vi "niWLAN - 80211abgnIQMeasurementsSettings.vi"(0 "niwlan analysis session":T6, 1 "WLAN Measurement Settings":T1={"OFDM Advanced Controls(11ag)"={"OFDM Auto Compute Acquisition Length Enabled"=0, "OFDM Maximum Symbols Used"=0, "OFDM Time Tracking Enabled"=0, "OFDM Channel Tracking Enabled"=0, "OFDM Amplitude Tracking Enabled"=1, "OFDM CFO Estimation Method"=0, "OFDM Phase Tracking Method"=0, "OFDM Header Detection Enabled"=0, "OFDM MAC FCS Check Enabled"=0, "#Avg"=10, "#Iterations"=10}, "DSSS Demod Parameters"={"DSSS Auto Compute Acquisition Length Enabled"=0, "DSSS Equalization Enabled"=0, "DSSS Header Detection Enabled"=0, "DSSS MAC FCS Check Enabled"=0, "DSSS Measurement Start Location"=0, "DSSS Phase Tracking Method"=0, "DSSS Maximum Chips Used"=0, "DSSS Reference Pulse Shaping Filter"=0, "DSSS Reference Pulse Shaping Filter Coefficient"=0.0, "# Avg"=1024, "# Iterations"=1024, "DSSS Power Ramp Enabled"=0}, "OFDM Advanced Controls (11n)"={"OFDM Auto Compute Acquisition Length Enabled"=0, "OFDM Maximum Symbols Used"=0, "OFDM Time Tracking Enabled"=0, "OFDM Channel Tracking Enabled"=0, "OFDM Amplitude Tracking Enabled"=1, "OFDM CFO Estimation Method"=0, "OFDM Phase Tracking Method"=0, "OFDM Header Detection Enabled"=0, "OFDM MAC FCS Check Enabled"=0, "#Avg"=10, "#Iterations"=10}, "OFDM Advanced Controls(11ac)"={"OFDM Auto Compute Acquisition Length Enabled"=0, "OFDM Maximum Symbols Used"=0, "OFDM Time Tracking Enabled"=1, "OFDM Channel Tracking Enabled"=0, "OFDM Amplitude Tracking Enabled"=0, "OFDM CFO Estimation Method"=0, "OFDM Phase Tracking Method"=0, "OFDM Header Detection Enabled"=0, "OFDM MAC FCS Check Enabled"=0, "#Avg"=10, "#Iterations"=10}} {"OFDM Advanced Controls(11ac)"."OFDM Phase Tracking Method" items=["Standard", "Instantaneous", "None", "Standard with Cubic Spline Fit"]; "OFDM Advanced Controls(11ac)"."OFDM CFO Estimation Method" items=["Preamble Only", "Preamble and Data"]; "OFDM Advanced Controls(11ac)"."OFDM Channel Tracking Enabled" items=["False", "True"]; "OFDM Advanced Controls(11ac)"."OFDM Amplitude Tracking Enabled" items=["False", "True"]; "OFDM Advanced Controls(11ac)"."OFDM Time Tracking Enabled" items=["True"=1, "False"=0]; "OFDM Advanced Controls(11ac)"."OFDM Auto Compute Acquisition Length Enabled" items=["False", "True"]; "OFDM Advanced Controls(11ac)"."OFDM MAC FCS Check Enabled" items=["False", "True"]; "OFDM Advanced Controls(11ac)"."OFDM Header Detection Enabled" items=["False", "True"]; "OFDM Advanced Controls (11n)"."OFDM Phase Tracking Method" items=["Standard", "Instantaneous", "None", "Standard with Cubic Spline Fit"]; "OFDM Advanced Controls (11n)"."OFDM CFO Estimation Method" items=["Preamble Only", "Preamble and Data"]; "OFDM Advanced Controls (11n)"."OFDM Channel Tracking Enabled" items=["False", "True"]; "OFDM Advanced Controls (11n)"."OFDM Amplitude Tracking Enabled" items=["False", "True"]; "OFDM Advanced Controls (11n)"."OFDM Time Tracking Enabled" items=["True"=1, "False"=0]; "OFDM Advanced Controls (11n)"."OFDM Auto Compute Acquisition Length Enabled" items=["False", "True"]; "OFDM Advanced Controls (11n)"."OFDM MAC FCS Check Enabled" items=["False", "True"]; "OFDM Advanced Controls (11n)"."OFDM Header Detection Enabled" items=["False", "True"]; "DSSS Demod Parameters"."DSSS Power Ramp Enabled" items=["False", "True"]; "DSSS Demod Parameters"."DSSS Auto Compute Acquisition Length Enabled" items=["False", "True"]; "DSSS Demod Parameters"."DSSS Phase Tracking Method" items=["Standard", "Instantaneous"]; "DSSS Demod Parameters"."DSSS Equalization Enabled" items=["False", "True"]; "DSSS Demod Parameters"."DSSS Reference Pulse Shaping Filter" items=["Rectangular", "Raised Cosine", "Root Raised Cosine", "Gaussian"]; "DSSS Demod Parameters"."DSSS MAC FCS Check Enabled" items=["False", "True"]; "DSSS Demod Parameters"."DSSS Header Detection Enabled" items=["False", "True"]; "OFDM Advanced Controls(11ag)"."OFDM Phase Tracking Method" items=["Standard", "Instantaneous", "None", "Standard with Cubic Spline Fit"]; "OFDM Advanced Controls(11ag)"."OFDM CFO Estimation Method" items=["Preamble Only", "Preamble and Data"]; "OFDM Advanced Controls(11ag)"."OFDM Channel Tracking Enabled" items=["False", "True"]; "OFDM Advanced Controls(11ag)"."OFDM Amplitude Tracking Enabled" items=["False", "True"]; "OFDM Advanced Controls(11ag)"."OFDM Time Tracking Enabled" items=["True"=1, "False"=0]; "OFDM Advanced Controls(11ag)"."OFDM Auto Compute Acquisition Length Enabled" items=["False", "True"]; "OFDM Advanced Controls(11ag)"."OFDM MAC FCS Check Enabled" items=["False", "True"]; "OFDM Advanced Controls(11ag)"."OFDM Header Detection Enabled" items=["False", "True"]}, 2 "Measurement Type":T4(ring), 5 "TV Parameters(DataType)":T5 {"Standard" items=["80211A/G/J/P OFDM", "80211B/G DSSS", "80211G DSSSOFDM", "80211N MIMOOFDM", "80211AC MIMOOFDM"]; "OFDM Data Rate (Mbps)" items=["6", "9", "12", "18", "24", "36", "48", "54"]; "80211n PLCP Frame Format" items=["Mixed Format", "Greenfield Format"]; "FEC Coding Type" items=["BCC", "LDPC"]; "DSSS Data Rate (Mbps)" items=["1", "2", "5.5 CCK", "5.5 PBCC", "11 CCK", "11 PBCC", "22", "33"]}, 7 "Set TV ?":bool, 11 "error in":errorcluster, 13 "Cal Routine ?":bool) -> (4 "niWLAN session":T6, 15 "error out":errorcluster)   [LabVIEW 2012]
uses:
  <vilib>/RF Toolkits/WLAN/analysis/controls/wlanv1 Analysis Refnum.ctl
  TV/RW/Includes/WLAN - TV - RW - INC - TV_DataType_Cluster.ctl
  TV/RW/Includes/WLAN - TV - RW - INC - Tx_Measurement_Cluster.ctl
  TV/RW/Includes/WLAN - TV - RW - INC - TV_OFDM Demod.ctl
  TV/RW/Includes/WLAN - TV - RW - INC - TV_DSSS Demod.ctl
  <resource>/objmgr/niWLANAnalysis.rc
panel:
  out "Standard":i32(ring) items=["80211A/G/J/P OFDM", "80211B/G DSSS", "80211G DSSSOFDM", "80211N MIMOOFDM", "80211AC MIMOOFDM"]
  # "Hardware Configuration"
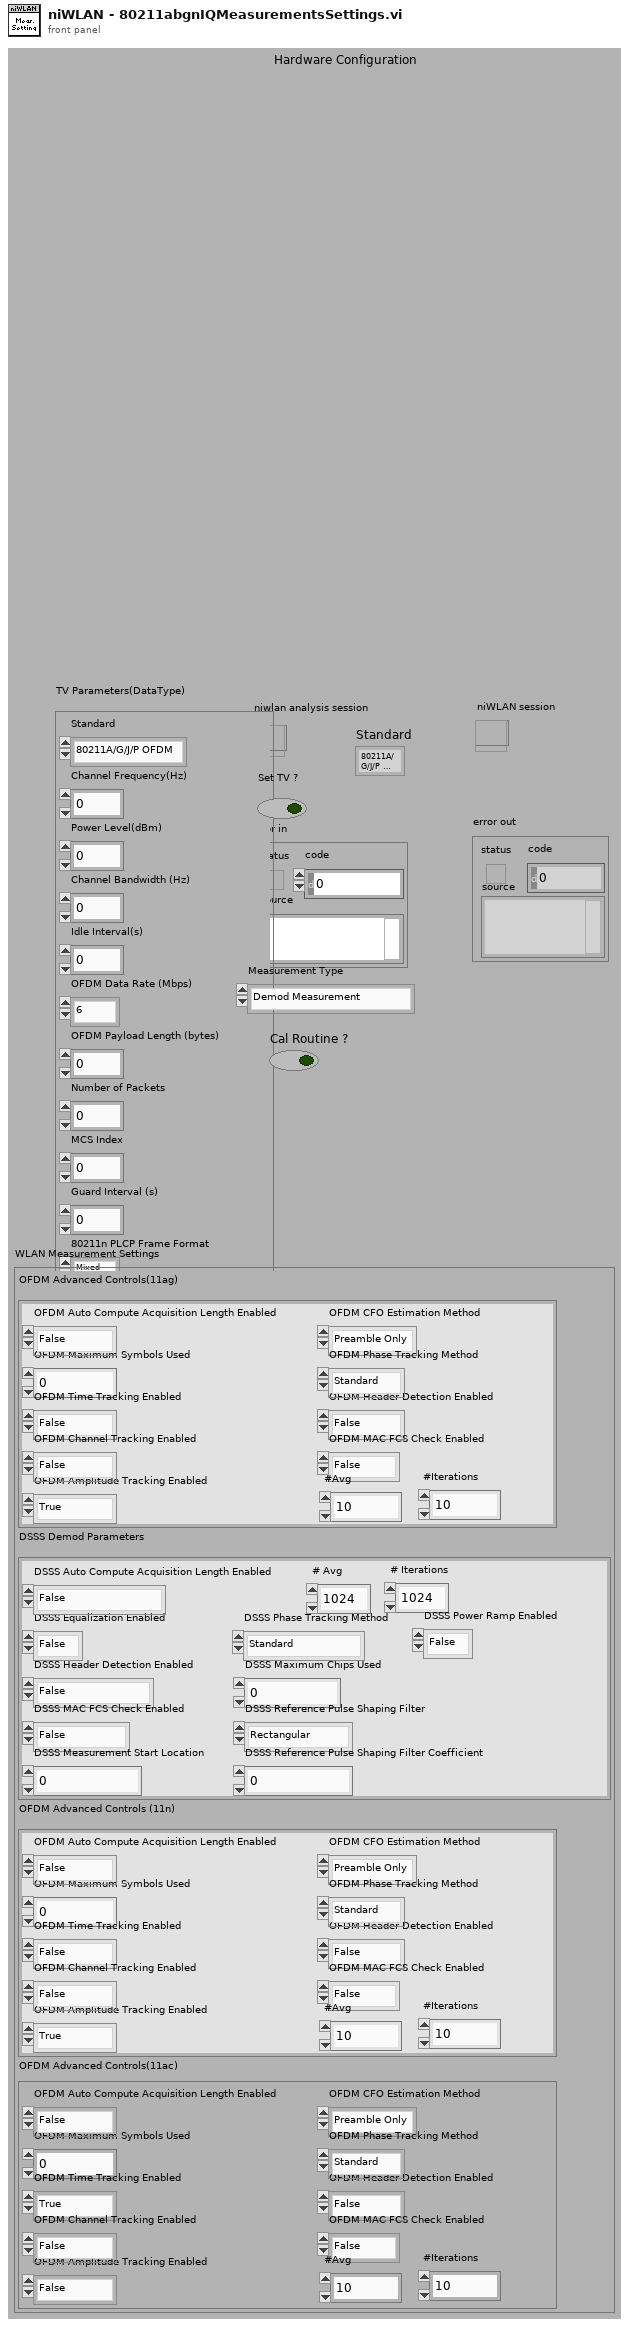
[diagram p1: front panel]
types:
  T1 = typedef "WLAN - TV - RW - INC - Tx_Measurement_Cluster.ctl" = cluster{"OFDM Advanced Controls(11ag)":T2, "DSSS Demod Parameters":T3, "OFDM Advanced Controls (11n)":T2, "OFDM Advanced Controls(11ac)":cluster{"OFDM Auto Compute Acquisition Length Enabled":i32, "OFDM Maximum Symbols Used":i32, "OFDM Time Tracking Enabled":i32, "OFDM Channel Tracking Enabled":i32, "OFDM Amplitude Tracking Enabled":i32, "OFDM CFO Estimation Method":i32, "OFDM Phase Tracking Method":i32, "OFDM Header Detection Enabled":i32, "OFDM MAC FCS Check Enabled":i32, "#Avg":i32, "#Iterations":i32}}
  T2 = typedef "WLAN - TV - RW - INC - TV_OFDM Demod.ctl" = cluster{"OFDM Auto Compute Acquisition Length Enabled":i32, "OFDM Maximum Symbols Used":i32, "OFDM Time Tracking Enabled":i32, "OFDM Channel Tracking Enabled":i32, "OFDM Amplitude Tracking Enabled":i32, "OFDM CFO Estimation Method":i32, "OFDM Phase Tracking Method":i32, "OFDM Header Detection Enabled":i32, "OFDM MAC FCS Check Enabled":i32, "#Avg":i32, "#Iterations":i32}
  T3 = typedef "WLAN - TV - RW - INC - TV_DSSS Demod.ctl" = cluster{"DSSS Auto Compute Acquisition Length Enabled":i32, "DSSS Equalization Enabled":i32, "DSSS Header Detection Enabled":i32, "DSSS MAC FCS Check Enabled":i32, "DSSS Measurement Start Location":i32, "DSSS Phase Tracking Method":i32, "DSSS Maximum Chips Used":i32, "DSSS Reference Pulse Shaping Filter":i32, "DSSS Reference Pulse Shaping Filter Coefficient":dbl, "# Avg":i32, "# Iterations":i32, "DSSS Power Ramp Enabled":i32}
  T4 = enum16{"Demod Measurement", "Spectrum Measurement"}
  T5 = typedef "WLAN - TV - RW - INC - TV_DataType_Cluster.ctl" = cluster{"Standard":i32, "Channel Frequency(Hz)":dbl, "Power Level(dBm)":dbl, "Channel Bandwidth (Hz)":dbl, "Idle Interval(s)":dbl, "OFDM Data Rate (Mbps)":i32, "OFDM Payload Length (bytes)":i32, "Number of Packets":i32, "MCS Index":i32, "Guard Interval (s)":dbl, "80211n PLCP Frame Format":i32, "FEC Coding Type":i32, "DSSS Data Rate (Mbps)":i32, "DSSS Payload Length (bytes)":i32, "N_SS":i32}
  T6 = typedef "wlanv1 Analysis Refnum.ctl" = refnum<k20>
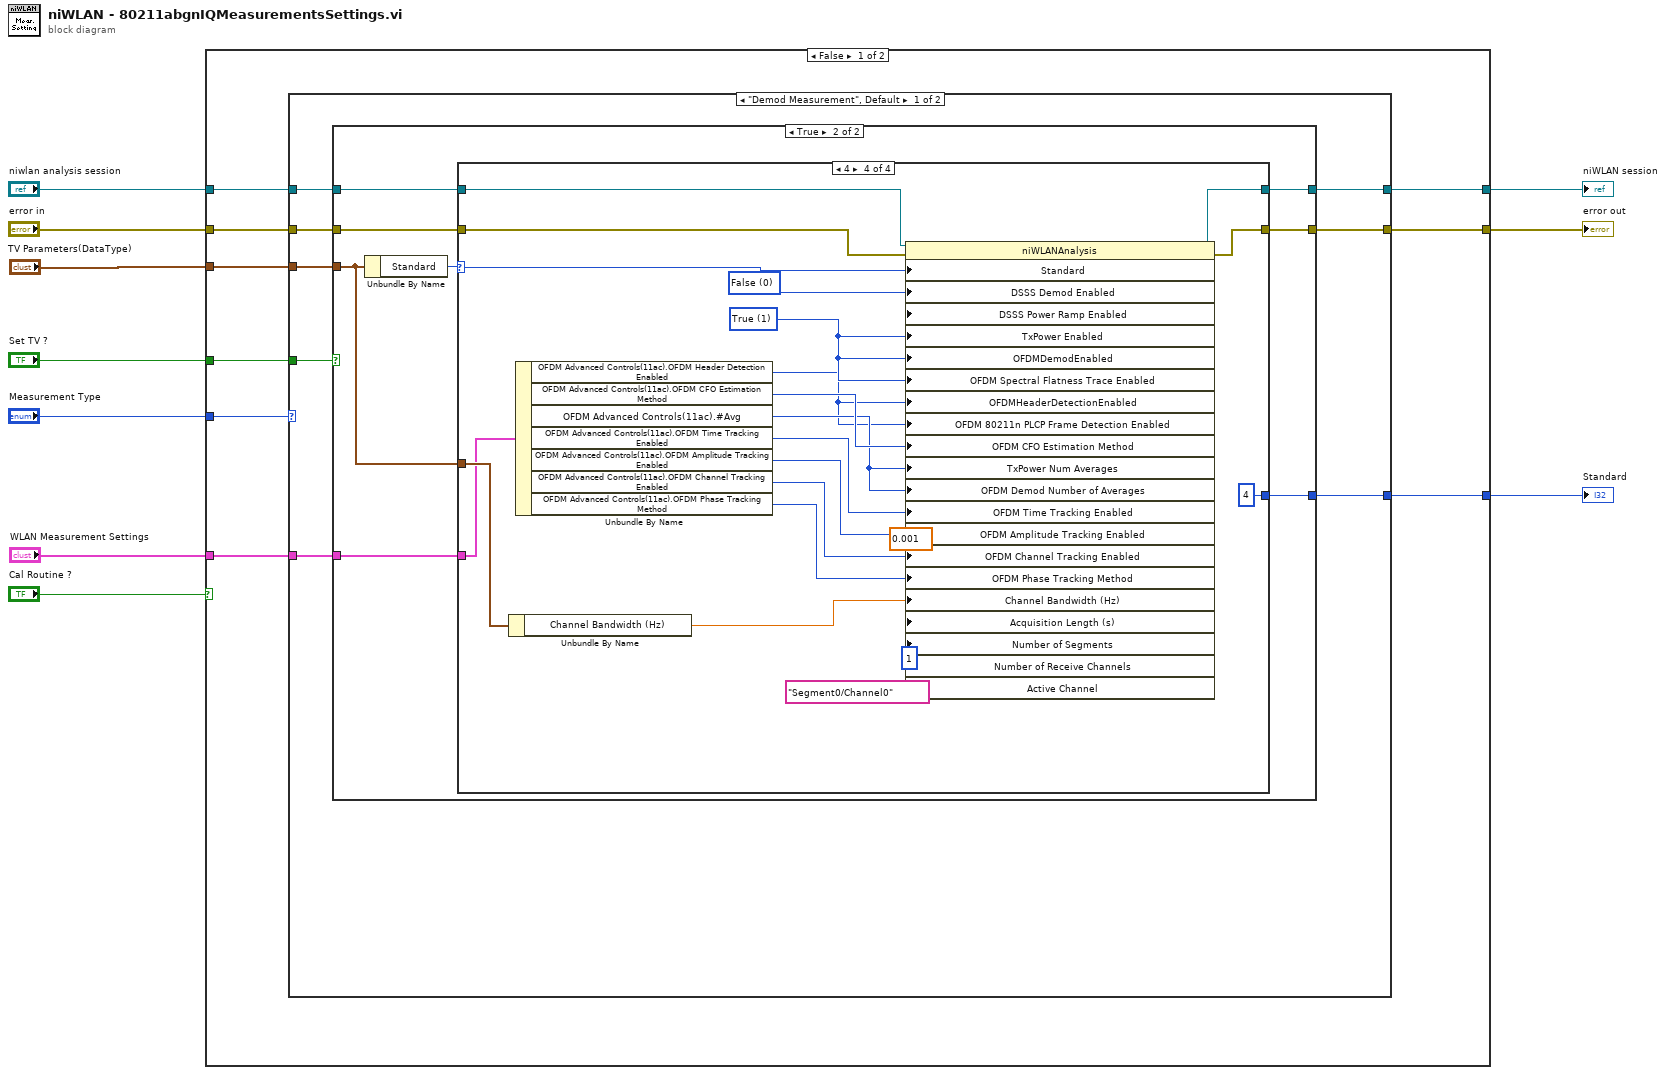
[diagram p0: block diagram]
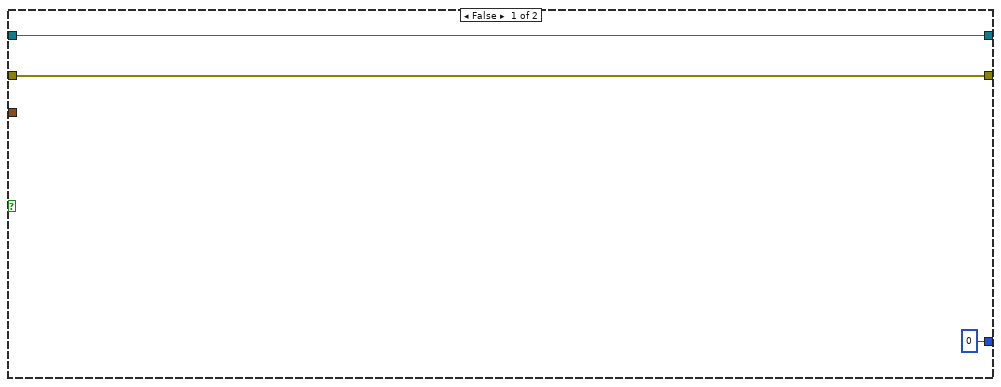
[diagram p2: hidden frame]
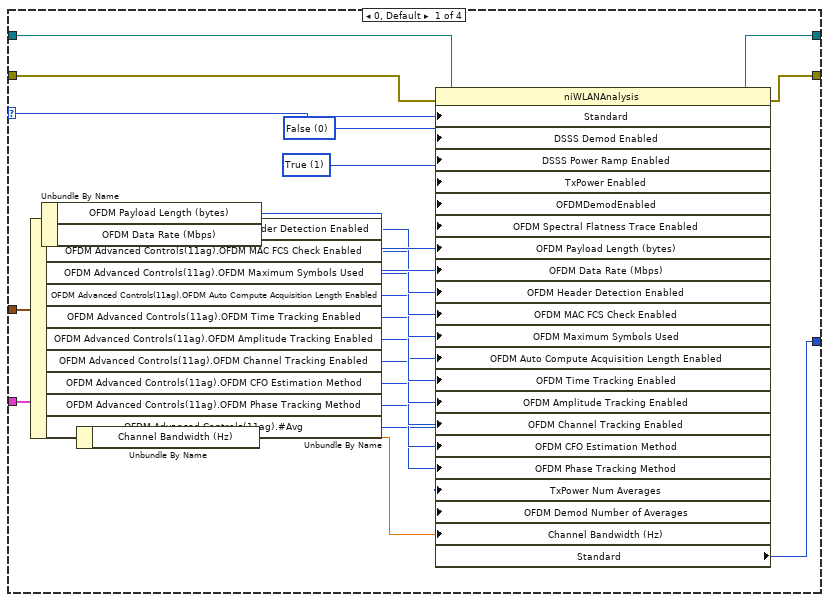
[diagram p3: hidden frame]
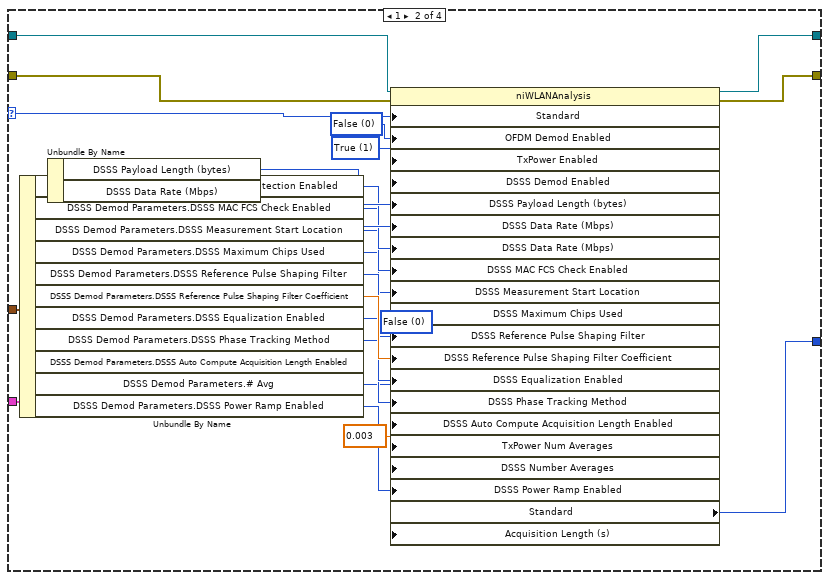
[diagram p4: hidden frame]
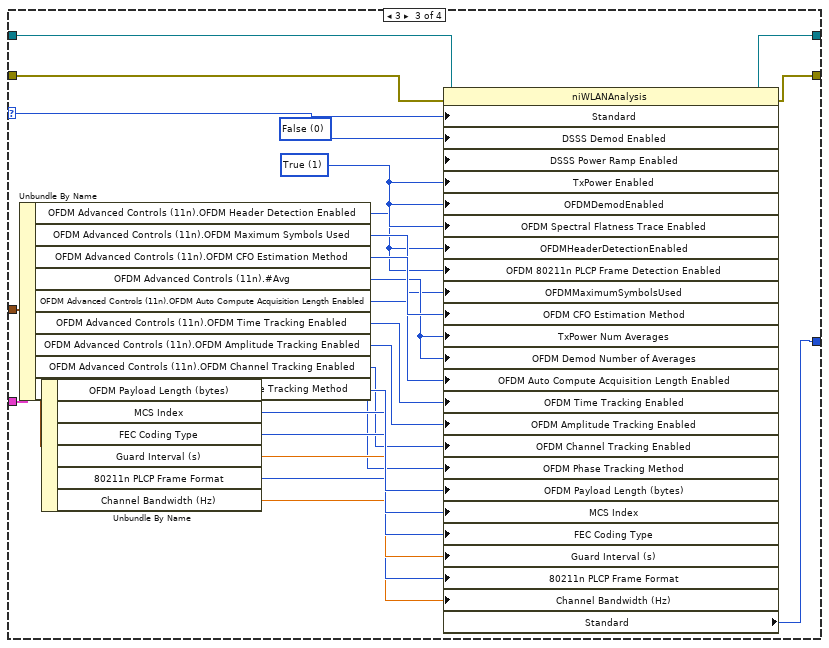
[diagram p5: hidden frame]
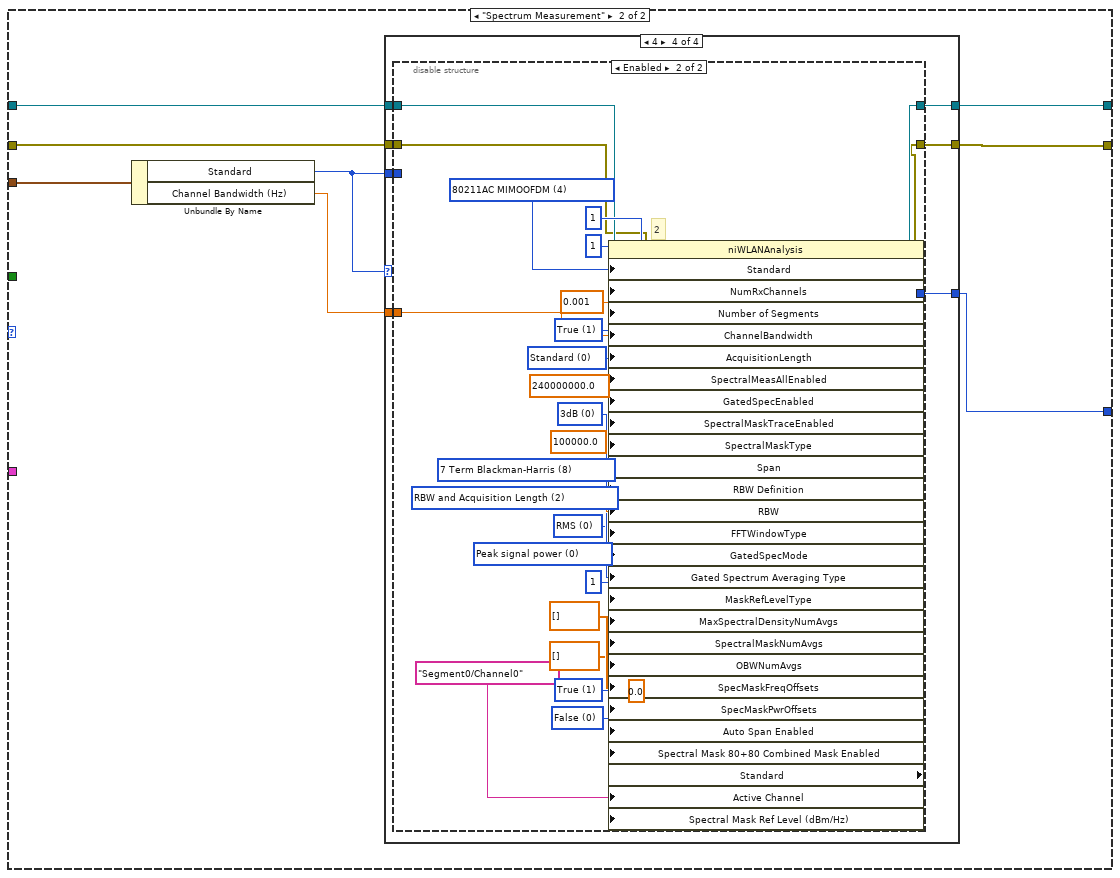
[diagram p6: hidden frame]
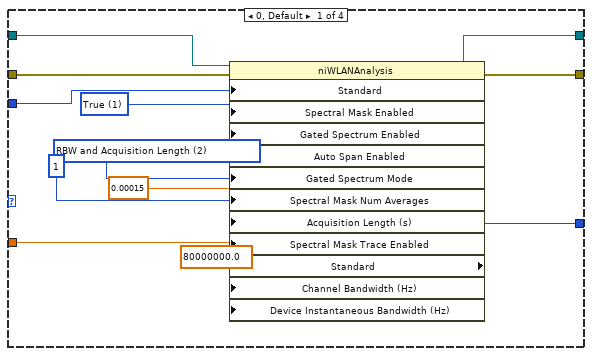
[diagram p7: hidden frame]
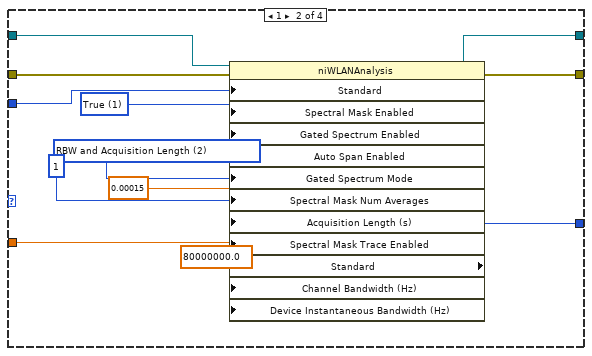
[diagram p8: hidden frame]
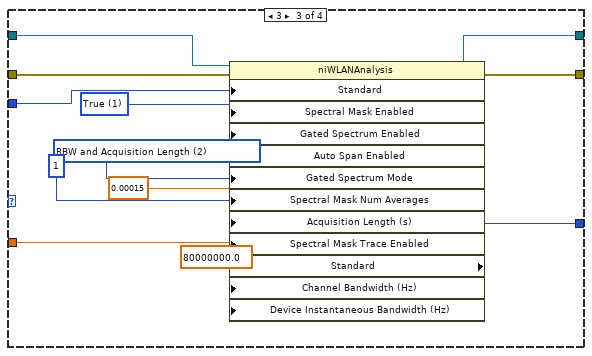
[diagram p9: hidden frame]
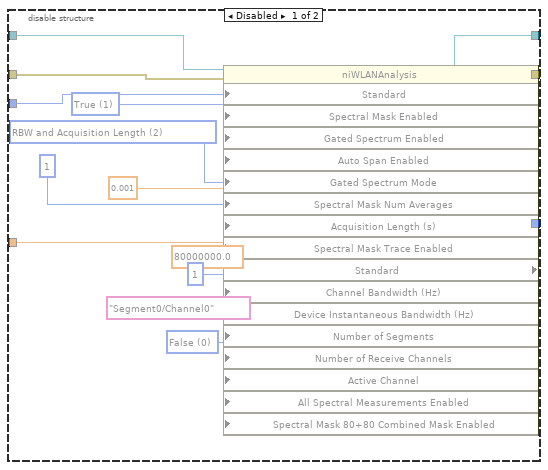
[diagram p10: hidden frame]
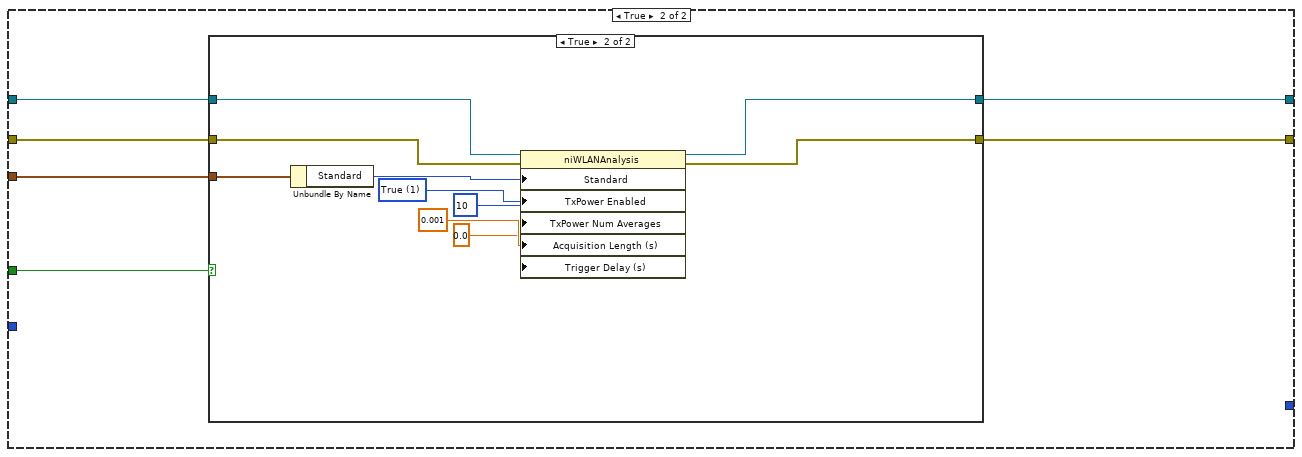
[diagram p11: hidden frame]
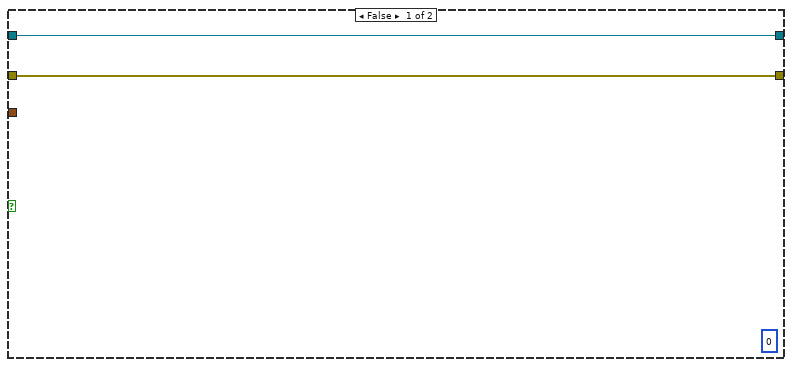
[diagram p12: hidden frame]
diagram:
  n1 = case shown="False" "Cal Routine ?" {
    tunnel: "niwlan analysis session" -> [w19 w229]
    tunnel: "error in" -> [w18 w228]
    tunnel: [w17 w227] -> w8
    tunnel: [w16 w226] -> w7
    tunnel: "TV Parameters(DataType)" -> [w15 w225]
    tunnel: "Set TV ?" -> [w14 w224]
    tunnel: "Measurement Type" -> [w13 _]
    tunnel: [w12 _] -> w3
    tunnel: "WLAN Measurement Settings" -> [w11 _]
    frame False {
      n2 = case shown="\"Demod Measurement\", Default" w13 {
        tunnel: w19 -> [w27 w139]
        tunnel: w18 -> [w26 w138]
        tunnel: [w25 w136] -> w17
        tunnel: [w24 w135] -> w16
        tunnel: w15 -> [w23 w137]
        tunnel: w14 -> [w22 _]
        tunnel: [w21 w134] -> w12
        tunnel: w11 -> [w20 _]
        frame "Demod Measurement", Default {
          n3 = case shown="True" w22 {
            tunnel: w27 -> [w30 w38]
            tunnel: w26 -> [w29 w37]
            tunnel: [w30 w36] -> w25
            tunnel: [w29 w35] -> w24
            tunnel: w23 -> [_ w33]
            tunnel: [0 ("Standard") w32] -> w21
            tunnel: w20 -> [_ w31]
            frame False {
            }
            frame True {
              n4 = Unbundle By Name(w33) -> ("Standard"=w34:i32)
              n5 = case shown="4" w34 {
                selector: w34 -> [w57 w81 w106 w127]
                tunnel: w38 -> [w61 w85 w110 w131]
                tunnel: w37 -> [w60 w84 w109 w130]
                tunnel: [w59 w83 w108 w129] -> w36
                tunnel: [w58 w82 w107 w128] -> w35
                tunnel: w33 -> [w43 w80 w105 w126]
                tunnel: [w41 w65 w98 4 ("Standard")] -> w32
                tunnel: w31 -> [w54 w75 w97 w124]
                frame 0, Default {
                  w39 = 0 items=["False", "True"] ("DSSS Demod Enabled")
                  w53 = 1 items=["False", "True"] ("OFDMDemodEnabled")
                  n6 = Unbundle By Name(w54) -> ("OFDM Advanced Controls(11ag).OFDM Header Detection Enabled"=w52:i32, "OFDM Advanced Controls(11ag).OFDM MAC FCS Check Enabled"=w51:i32, "OFDM Advanced Controls(11ag).OFDM Maximum Symbols Used"=w50:i32, "OFDM Advanced Controls(11ag).OFDM Auto Compute Acquisition Length Enabled"=w40:i32, "OFDM Advanced Controls(11ag).OFDM Time Tracking Enabled"=w49:i32, "OFDM Advanced Controls(11ag).OFDM Amplitude Tracking Enabled"=w48:i32, "OFDM Advanced Controls(11ag).OFDM Channel Tracking Enabled"=w47:i32, "OFDM Advanced Controls(11ag).OFDM CFO Estimation Method"=w46:i32, "OFDM Advanced Controls(11ag).OFDM Phase Tracking Method"=w45:i32, "OFDM Advanced Controls(11ag).#Avg"=w44:i32)
                  n7 = Unbundle By Name(w43) -> ("OFDM Payload Length (bytes)"=w56:i32, "OFDM Data Rate (Mbps)"=w55:i32)
                  n8 = Unbundle By Name(w43) -> ("Channel Bandwidth (Hz)"=w42:dbl)
                  n9 = property class="niWLANAnalysis"(reference=w61, error in=w60, "Standard"=w57, "DSSS Demod Enabled"=w39, "DSSS Power Ramp Enabled"=w39, "TxPower Enabled"=w53, "OFDMDemodEnabled"=w53, "OFDM Spectral Flatness Trace Enabled"=w53, "OFDM Payload Length (bytes)"=w56, "OFDM Data Rate (Mbps)"=w55, "OFDM Header Detection Enabled"=w52, "OFDM MAC FCS Check Enabled"=w51, "OFDM Maximum Symbols Used"=w50, "OFDM Auto Compute Acquisition Length Enabled"=w40, "OFDM Time Tracking Enabled"=w49, "OFDM Amplitude Tracking Enabled"=w48, "OFDM Channel Tracking Enabled"=w47, "OFDM CFO Estimation Method"=w46, "OFDM Phase Tracking Method"=w45, "TxPower Num Averages"=w44, "OFDM Demod Number of Averages"=w44, "Channel Bandwidth (Hz)"=w42) -> (reference out=w59:T6, error out=w58:errorcluster, "Standard"=w41:i32)
                }
                frame 1 {
                  w63 = 0 items=["False", "True"] ("DSSS Auto Compute Acquisition Length Enabled")
                  w76 = 0 items=["False", "True"] ("OFDM Demod Enabled")
                  w77 = 1 items=["False", "True"] ("OFDMDemodEnabled")
                  n10 = Unbundle By Name(w75) -> ("DSSS Demod Parameters.DSSS Header Detection Enabled"=w72:i32, "DSSS Demod Parameters.DSSS MAC FCS Check Enabled"=w71:i32, "DSSS Demod Parameters.DSSS Measurement Start Location"=w70:i32, "DSSS Demod Parameters.DSSS Maximum Chips Used"=w69:i32, "DSSS Demod Parameters.DSSS Reference Pulse Shaping Filter"=w73:i32, "DSSS Demod Parameters.DSSS Reference Pulse Shaping Filter Coefficient"=w74:dbl, "DSSS Demod Parameters.DSSS Equalization Enabled"=w68:i32, "DSSS Demod Parameters.DSSS Phase Tracking Method"=w67:i32, "DSSS Demod Parameters.# Avg"=w66:i32, "DSSS Demod Parameters.DSSS Power Ramp Enabled"=w64:i32)  [unwired: 1 out]
                  n11 = Unbundle By Name(w80) -> ("DSSS Payload Length (bytes)"=w79:i32, "DSSS Data Rate (Mbps)"=w78:i32)
                  n12 = property class="niWLANAnalysis"(reference=w85, error in=w84, "Standard"=w81, "OFDM Demod Enabled"=w76, "TxPower Enabled"=w77, "DSSS Demod Enabled"=w77, "DSSS Payload Length (bytes)"=w79, "DSSS Data Rate (Mbps)"=w78, "DSSS Data Rate (Mbps)"=w72, "DSSS MAC FCS Check Enabled"=w71, "DSSS Measurement Start Location"=w70, "DSSS Maximum Chips Used"=w69, "DSSS Reference Pulse Shaping Filter"=w73, "DSSS Reference Pulse Shaping Filter Coefficient"=w74, "DSSS Equalization Enabled"=w68, "DSSS Phase Tracking Method"=w67, "DSSS Auto Compute Acquisition Length Enabled"=w63, "TxPower Num Averages"=w66, "DSSS Number Averages"=w66, "DSSS Power Ramp Enabled"=w64, "Acquisition Length (s)"=0.003) -> (reference out=w83:T6, error out=w82:errorcluster, "Standard"=w65:i32)
                }
                frame 3 {
                  w86 = 0 items=["False", "True"] ("OFDMDemodEnabled")
                  w90 = 1 items=["False", "True"] ("OFDMDemodEnabled")
                  n13 = Unbundle By Name(w97) -> ("OFDM Advanced Controls (11n).OFDM Header Detection Enabled"=w87:i32, "OFDM Advanced Controls (11n).OFDM Maximum Symbols Used"=w88:i32, "OFDM Advanced Controls (11n).OFDM CFO Estimation Method"=w96:i32, "OFDM Advanced Controls (11n).#Avg"=w89:i32, "OFDM Advanced Controls (11n).OFDM Auto Compute Acquisition Length Enabled"=w95:i32, "OFDM Advanced Controls (11n).OFDM Time Tracking Enabled"=w94:i32, "OFDM Advanced Controls (11n).OFDM Amplitude Tracking Enabled"=w93:i32, "OFDM Advanced Controls (11n).OFDM Channel Tracking Enabled"=w92:i32, "OFDM Advanced Controls (11n).OFDM Phase Tracking Method"=w91:i32)
                  n14 = Unbundle By Name(w105) -> ("OFDM Payload Length (bytes)"=w104:i32, "MCS Index"=w103:i32, "FEC Coding Type"=w102:i32, "Guard Interval (s)"=w101:dbl, "80211n PLCP Frame Format"=w100:i32, "Channel Bandwidth (Hz)"=w99:dbl)
                  n15 = property class="niWLANAnalysis"(reference=w110, error in=w109, "Standard"=w106, "DSSS Demod Enabled"=w86, "DSSS Power Ramp Enabled"=w86, "TxPower Enabled"=w90, "OFDMDemodEnabled"=w90, "OFDM Spectral Flatness Trace Enabled"=w90, "OFDMHeaderDetectionEnabled"=w87, "OFDM 80211n PLCP Frame Detection Enabled"=w87, "OFDMMaximumSymbolsUsed"=w88, "OFDM CFO Estimation Method"=w96, "TxPower Num Averages"=w89, "OFDM Demod Number of Averages"=w89, "OFDM Auto Compute Acquisition Length Enabled"=w95, "OFDM Time Tracking Enabled"=w94, "OFDM Amplitude Tracking Enabled"=w93, "OFDM Channel Tracking Enabled"=w92, "OFDM Phase Tracking Method"=w91, "OFDM Payload Length (bytes)"=w104, "MCS Index"=w103, "FEC Coding Type"=w102, "Guard Interval (s)"=w101, "80211n PLCP Frame Format"=w100, "Channel Bandwidth (Hz)"=w99) -> (reference out=w108:T6, error out=w107:errorcluster, "Standard"=w98:i32)
                }
                frame 4 {
                  w114 = 1 ("Number of Segments")
                  w115 = 0 items=["False", "True"] ("OFDMDemodEnabled")
                  w118 = 1 items=["False", "True"] ("OFDMDemodEnabled")
                  n16 = Unbundle By Name(w126) -> ("Channel Bandwidth (Hz)"=w125:dbl)
                  n17 = Unbundle By Name(w124) -> ("OFDM Advanced Controls(11ac).OFDM Header Detection Enabled"=w116:i32, "OFDM Advanced Controls(11ac).OFDM CFO Estimation Method"=w123:i32, "OFDM Advanced Controls(11ac).#Avg"=w117:i32, "OFDM Advanced Controls(11ac).OFDM Time Tracking Enabled"=w122:i32, "OFDM Advanced Controls(11ac).OFDM Amplitude Tracking Enabled"=w121:i32, "OFDM Advanced Controls(11ac).OFDM Channel Tracking Enabled"=w120:i32, "OFDM Advanced Controls(11ac).OFDM Phase Tracking Method"=w119:i32)
                  n18 = property class="niWLANAnalysis"(reference=w131, error in=w130, "Standard"=w127, "DSSS Demod Enabled"=w115, "DSSS Power Ramp Enabled"=w115, "TxPower Enabled"=w118, "OFDMDemodEnabled"=w118, "OFDM Spectral Flatness Trace Enabled"=w118, "OFDMHeaderDetectionEnabled"=w116, "OFDM 80211n PLCP Frame Detection Enabled"=w116, "OFDM CFO Estimation Method"=w123, "TxPower Num Averages"=w117, "OFDM Demod Number of Averages"=w117, "OFDM Time Tracking Enabled"=w122, "OFDM Amplitude Tracking Enabled"=w121, "OFDM Channel Tracking Enabled"=w120, "OFDM Phase Tracking Method"=w119, "Channel Bandwidth (Hz)"=w125, "Acquisition Length (s)"=0.001, "Number of Segments"=w114, "Number of Receive Channels"=w114, "Active Channel"="Segment0/Channel0") -> (reference out=w129:T6, error out=w128:errorcluster)
                }
              }
            }
          }
        }
        frame "Spectrum Measurement" {
          n19 = Unbundle By Name(w137) -> ("Standard"=w132:i32, "Channel Bandwidth (Hz)"=w133:dbl)
          n20 = case shown="4" w132 {
            tunnel: w139 -> [w151 w163 w175 w182]
            tunnel: w138 -> [w150 w162 w174 w181]
            tunnel: [w149 w161 w173 w180] -> w136
            tunnel: [w148 w160 w172 w179] -> w135
            tunnel: [w147 w159 w171 w178] -> w134
            tunnel: w132 -> [w146 w158 w170 w177]
            tunnel: w133 -> [w141 w153 w165 w176]
            frame 0, Default {
              w144 = 2 items=["RBW", "Acquisition Length", "RBW and Acquisition Length"] ("Gated Spectrum Mode")
              w142 = 1 items=["False", "True"] ("OFDMDemodEnabled")
              n21 = property class="niWLANAnalysis"(reference=w151, error in=w150, "Standard"=w146, "Spectral Mask Enabled"=w142, "Gated Spectrum Enabled"=w142, "Auto Span Enabled"=w142, "Gated Spectrum Mode"=w144, "Spectral Mask Num Averages"=1 ("Averages"), "Acquisition Length (s)"=0.00015, "Spectral Mask Trace Enabled"=w142, "Channel Bandwidth (Hz)"=w141, "Device Instantaneous Bandwidth (Hz)"=80000000.0) -> (reference out=w149:T6, error out=w148:errorcluster, "Standard"=w147:i32)
            }
            frame 1 {
              w156 = 2 items=["RBW", "Acquisition Length", "RBW and Acquisition Length"] ("Gated Spectrum Mode")
              w154 = 1 items=["False", "True"] ("OFDMDemodEnabled")
              n22 = property class="niWLANAnalysis"(reference=w163, error in=w162, "Standard"=w158, "Spectral Mask Enabled"=w154, "Gated Spectrum Enabled"=w154, "Auto Span Enabled"=w154, "Gated Spectrum Mode"=w156, "Spectral Mask Num Averages"=1 ("Averages"), "Acquisition Length (s)"=0.00015, "Spectral Mask Trace Enabled"=w154, "Channel Bandwidth (Hz)"=w153, "Device Instantaneous Bandwidth (Hz)"=80000000.0) -> (reference out=w161:T6, error out=w160:errorcluster, "Standard"=w159:i32)
            }
            frame 3 {
              w168 = 2 items=["RBW", "Acquisition Length", "RBW and Acquisition Length"] ("Gated Spectrum Mode")
              w166 = 1 items=["False", "True"] ("OFDMDemodEnabled")
              n23 = property class="niWLANAnalysis"(reference=w175, error in=w174, "Standard"=w170, "Spectral Mask Enabled"=w166, "Gated Spectrum Enabled"=w166, "Auto Span Enabled"=w166, "Gated Spectrum Mode"=w168, "Spectral Mask Num Averages"=1 ("Averages"), "Acquisition Length (s)"=0.00015, "Spectral Mask Trace Enabled"=w166, "Channel Bandwidth (Hz)"=w165, "Device Instantaneous Bandwidth (Hz)"=80000000.0) -> (reference out=w173:T6, error out=w172:errorcluster, "Standard"=w171:i32)
            }
            frame 4 {
              n24 = disable-structure shown="Enabled" {
                disable-tunnel: w182 -> [w197 w206]
                disable-tunnel: w181 -> [w196 w203]
                disable-tunnel: [w195 w205] -> w180
                disable-tunnel: [w194 w204] -> w179
                disable-tunnel: [w193 w201] -> w178
                disable-tunnel: w177 -> [w192 _]
                disable-tunnel: w176 -> [w188 w202]
                frame Disabled {
                  w183 = 0 items=["False", "True"] ("Spectral Mask 80+80 Combined Mask Enabled")
                  w186 = 1 ("Number of Segments")
                  w190 = 2 items=["RBW", "Acquisition Length", "RBW and Acquisition Length"] ("Gated Spectrum Mode")
                  w184 = 1 items=["False", "True"] ("OFDMDemodEnabled")
                  n25 = property class="niWLANAnalysis"(reference=w197, error in=w196, "Standard"=w192, "Spectral Mask Enabled"=w184, "Gated Spectrum Enabled"=w184, "Auto Span Enabled"=w184, "Gated Spectrum Mode"=w190, "Spectral Mask Num Averages"=1 ("Averages"), "Acquisition Length (s)"=0.001, "Spectral Mask Trace Enabled"=w184, "Channel Bandwidth (Hz)"=w188, "Device Instantaneous Bandwidth (Hz)"=80000000.0, "Number of Segments"=w186, "Number of Receive Channels"=w186, "Active Channel"="Segment0/Channel0", "All Spectral Measurements Enabled"=w184, "Spectral Mask 80+80 Combined Mask Enabled"=w183) -> (reference out=w195:T6, error out=w194:errorcluster, "Standard"=w193:i32)
                }
                frame Enabled {
                  w211 = 0 items=["True"=1, "False"=0] ("Combine 80+80 Mask Enabled")
                  w212 = 1 items=["False", "True"] ("Auto Span Enabled")
                  w222 = 1 ("Number of Averages")
                  w214 = 0 items=["Peak signal power", "User defined"] ("Mask Reference Level Type")
                  w207 = 0 items=["RMS", "Log"] ("Gated Spectrum Averaging Type")
                  w218 = 2 items=["RBW", "Acquisition Length", "RBW and Acquisition Length"] ("Gated Spectrum Mode")
                  w219 = 8 items=["Uniform", "Hanning", "Hamming", "Blackman-Harris", "Exact Blackman", "Blackman", "Flat Top", "4 Term Blackman-Harris", "7 Term Blackman-Harris", "Low Side Lobe"] ("FFT Window Type")
                  w221 = 0 items=["3dB", "6dB", "ENBW", "bin width"] ("RBW Definition")
                  w208 = 0 items=["Standard", "User defined", "Standard at 5GHz"] ("Spectral Mask Type")
                  w198 = 4 items=["80211A/G/J/P OFDM", "80211B/G DSSS", "80211G DSSSOFDM", "80211N MIMOOFDM", "80211AC MIMOOFDM"] ("Standard")
                  w223 = 1 items=["False", "True"] ("SpectralMeasAllEnabled")
                  # "2"
                  n26 = property class="niWLANAnalysis"(reference=w206, error in=w203, "Standard"=w198, "NumRxChannels"=1 ("Number of Receive Channel"), "Number of Segments"=1 ("No. of Segments"), "ChannelBandwidth"=w202, "AcquisitionLength"=0.001 ("Acquisition Length (s)"), "SpectralMeasAllEnabled"=w223, "GatedSpecEnabled"=w223, "SpectralMaskTraceEnabled"=w223, "SpectralMaskType"=w208, "Span"=240000000.0 ("Span (Hz)"), "RBW Definition"=w221, "RBW"=100000.0 ("RBW (Hz)"), "FFTWindowType"=w219, "GatedSpecMode"=w218, "Gated Spectrum Averaging Type"=w207, "MaskRefLevelType"=w214, "MaxSpectralDensityNumAvgs"=w222, "SpectralMaskNumAvgs"=w222, "OBWNumAvgs"=w222, "SpecMaskFreqOffsets"=dbl[] [] ("Spectral Mask Frequency Offset (Hz)"), "SpecMaskPwrOffsets"=dbl[] [] ("Spectral Mask Power Offset(dB)"), "Auto Span Enabled"=w212, "Spectral Mask 80+80 Combined Mask Enabled"=w211, "Active Channel"="Segment0/Channel0", "Spectral Mask Ref Level (dBm/Hz)"=0.0) -> (reference out=w205:T6, error out=w204:errorcluster, "Standard"=w201:i32)
                }
              }
            }
          }
        }
      }
    }
    frame True {
      n27 = case shown="True" w224 {
        tunnel: w229 -> [w231 w241]
        tunnel: w228 -> [w230 w240]
        tunnel: [w231 w239] -> w227
        tunnel: [w230 w238] -> w226
        tunnel: w225 -> [_ w236]
        frame False {
          (unwired) 0 ("Standard")
        }
        frame True {
          w233 = 1 items=["False", "True"] ("OFDMDemodEnabled")
          n28 = Unbundle By Name(w236) -> ("Standard"=w237:i32)
          n29 = property class="niWLANAnalysis"(reference=w241, error in=w240, "Standard"=w237, "TxPower Enabled"=w233, "TxPower Num Averages"=10, "Acquisition Length (s)"=0.001, "Trigger Delay (s)"=0.0 ("Trigger Delay (sec)")) -> (reference out=w239:T6, error out=w238:errorcluster)
        }
      }
    }
  }
  "error out" <- w7
  "niWLAN session" <- w8
  "Standard" <- w3
